vi "Init.vi"(8 "error in (no error)":errorcluster, 11 "FPGA in":refnum<class "FPGA.lvclass">) -> (0 "error out":errorcluster, 3 "FPGA out":refnum<class "FPGA.lvclass">)   [LabVIEW 2019, in "FPGA.lvclass"]
uses:
  FPGA.lvclass
  FPGA.lvclass/FPGA.ctl
  <vilib>/rvi/interface/common/niFpgaWaitOnOcc.vi
  <vilib>/Utility/error.llb/Error Cluster From Error Code.vi
  <vilib>/rvi/interface/nirviMethod/nirviMethod.xnode
  <vilib>/rvi/interface/nirviOpenFPGA/nirviOpenFPGA.xnode
  FPGA Bitfiles/hydrov2_FPGATarget_MAINFPGA_-K0CvU7hRyo.lvbitx
  FPGA/MAIN FPGA.vi
  <vilib>/FPGAPlugInAG/cRIO-9035/niLvFpga_Open_cRIO-9035.vi
  <vilib>/rvi/interface/common/dynamic/niFpgaDynamicAddResources.vi
  <vilib>/FPGAPlugInAG/Dynamic/niLvFpga_ConfigureFifo_Dynamic.vi
  <vilib>/rvi/errors/niLvFpgaMergeErrorWithErrorCode.vi
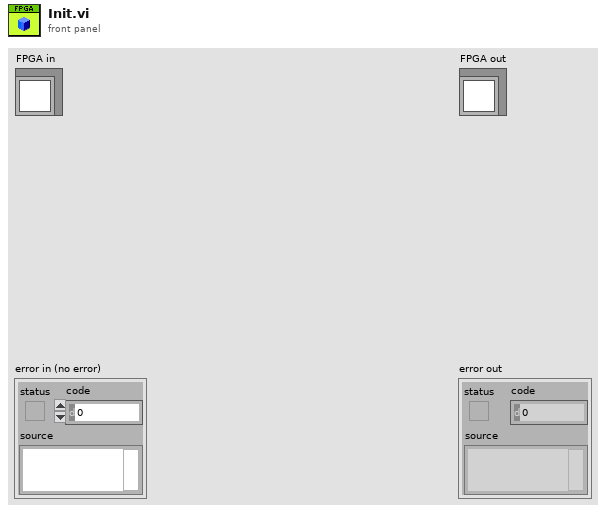
[diagram p1: front panel]
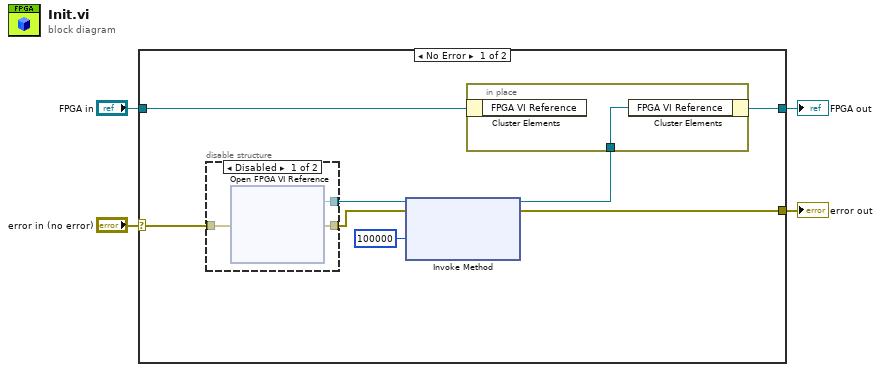
[diagram p0: block diagram]
diagram:
  n1 = case shown="No Error" "error in (no error)" {
    selector: "error in (no error)" -> [w12 w18]
    tunnel: [w5 w18] -> w3
    tunnel: [w9 w17] -> w1
    tunnel: "FPGA in" -> [w11 w17]
    frame No Error {
      n2 = disable-structure shown="Disabled" {
        disable-tunnel: [w16 _] -> w10
        disable-tunnel: [w15 _] -> w6
        disable-tunnel: w12 -> [w14 _]
        frame Disabled {
          n3 = xnode "Open FPGA VI Reference"("error in"=w14) -> ("FPGA VI Reference Out"=w16:refnum<k20>, "error out"=w15:errorcluster)  [unwired: 1 in]
        }
        frame Enabled {
        }
      }
      n4 = xnode "Invoke Method"("FPGA VI Reference In"=w10, "error in"=w6, "Requested Depth"=u32 100000) -> ("FPGA VI Reference Out"=w8:refnum<k20>, "error out"=w5:errorcluster)  [unwired: 1 out]
      n5 = in-place {
        in-place-border: w8 -> [w13]
        n6 = in-place-cluster #1(w11) -> ()  [unwired: 1 out]
        n7 = in-place-cluster #1("FPGA VI Reference"=w13) -> (w9:refnum<class "FPGA.lvclass">)
      }
    }
    frame Error {
    }
  }
  "error out" <- w3
  "FPGA out" <- w1
